vi "Compare_Data.vi"(8 "error in (no error)":errorcluster, 11 "String":string) -> (0 "error out":errorcluster, 3 "Boolean":bool)   [LabVIEW 2016]
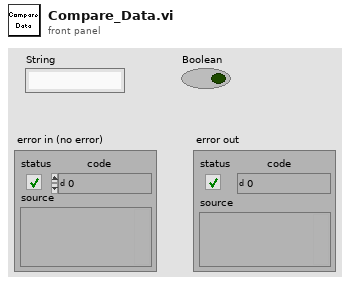
[diagram p1: front panel]
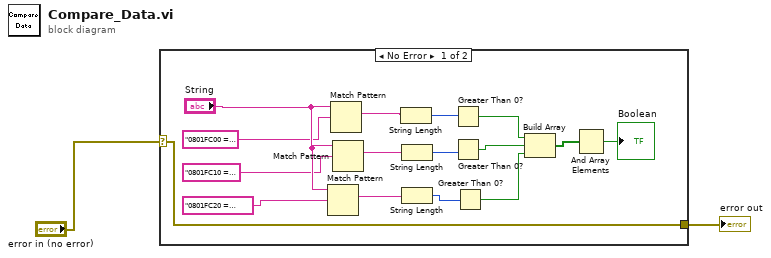
[diagram p0: block diagram]
diagram:
  n1 = case shown="No Error" "error in (no error)" {
    selector: "error in (no error)" -> [w3 w19]
    tunnel: [w3 w19] -> w1
    frame No Error {
      n2 = Match Pattern(string="String", regular expression="0801FC20 = 00006E69 00000001 00000006 00000000") -> (match substring=w10:string)  [unwired: 1 in, 3 out]
      n3 = Match Pattern(string="String", regular expression="0801FC00 = 72656D45 2D6E6F73 616C6F53 00004448") -> (match substring=w8:string)  [unwired: 1 in, 3 out]
      n4 = Match Pattern(string="String", regular expression="0801FC10 = 2D4D4353 746F6F42 64616F6C 622E7265") -> (match substring=w9:string)  [unwired: 1 in, 3 out]
      n5 = String Length(string=w8) -> (length=w11:i32)
      n6 = String Length(string=w9) -> (length=w12:i32)
      n7 = String Length(string=w10) -> (length=w13:i32)
      n8 = Greater Than 0?(x=w11) -> (x > 0?=w14:bool)
      n9 = Greater Than 0?(x=w12) -> (x > 0?=w15:bool)
      n10 = Greater Than 0?(x=w13) -> (x > 0?=w16:bool)
      n11 = Build Array(w14, w15, w16) -> (w17:bool[])
      n12 = And Array Elements(Boolean array=w17) -> (logical AND=→"Boolean":bool)
    }
    frame Error {
    }
  }
  "error out" <- w1
